vi "Bodies_GetPtJacobian.vi"(8 "error in (no error)":errorcluster, 10 "Point":T1, 11 "Bodies.lvclass":refnum<class "Bodies.lvclass">) -> (0 "error out":errorcluster, 1 "PointInGCS":dbl[](array[numeric]) format="%#.6f", 2 "Jacobian":dbl[][](array[numeric]) format="%#.6f", 3 "Bodies.lvclass 2":refnum<class "Bodies.lvclass">)   [LabVIEW 2015, in "Bodies.lvclass"]
doc: "Calculate velocity Jacobian v=[J] dq. Input the point of interest (POI) in local coordinate system. Output the Jacobian that transfers the joint speed to the POI's speed."
uses:
  Bodies.lvclass
  PointOnBody.ctl
  Bodies.lvclass/Bodies.ctl
  xyzO.ctl
  <vilib>/Analysis/NI_AALPro.lvlib
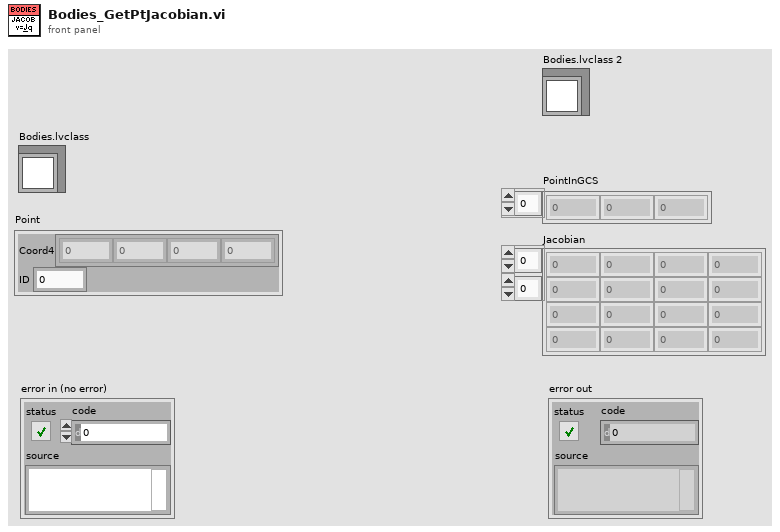
[diagram p1: front panel]
types:
  T1 = typedef "Bodies.lvclass/PointOnBody.ctl" = cluster{"Coord4":dbl[], "ID":i32}
  T2 = typedef "Bodies.lvclass/xyzO.ctl" = enum16{"X", "Y", "Z", "O"}
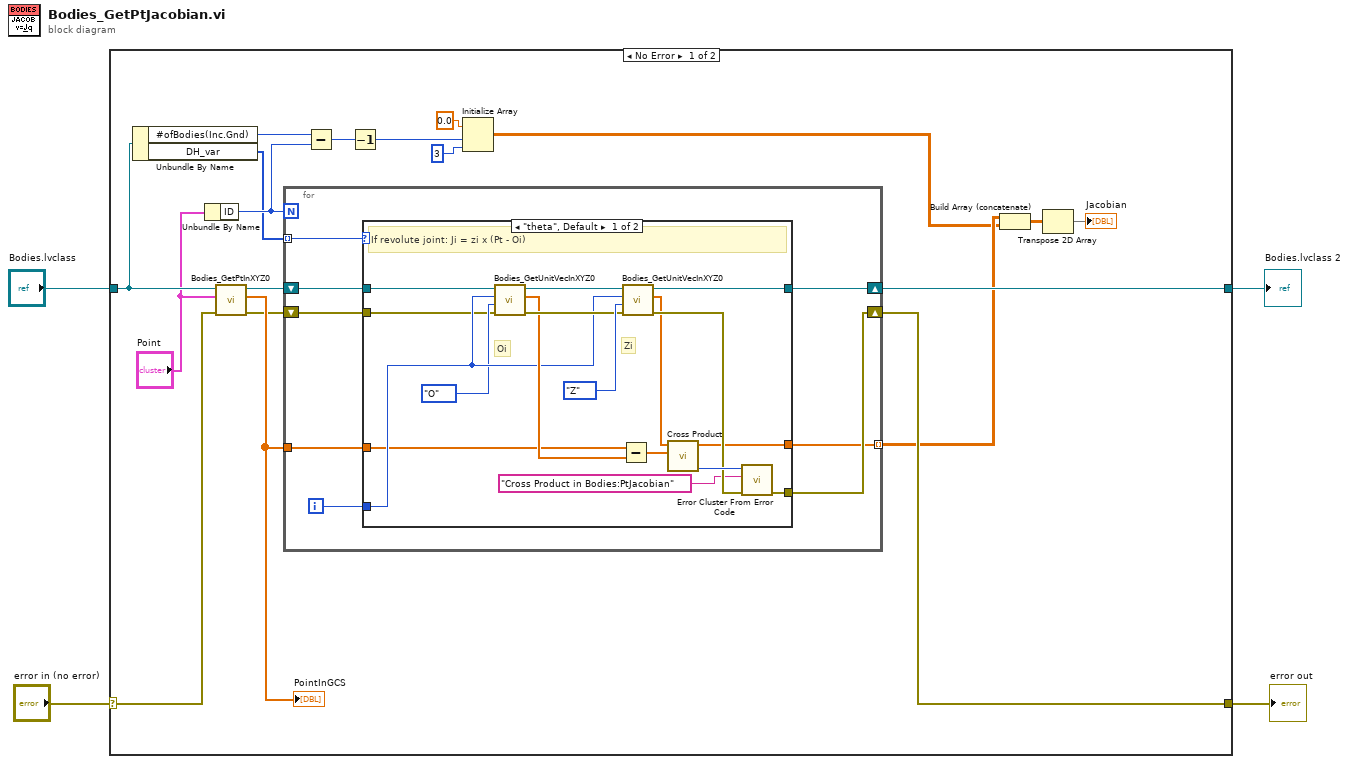
[diagram p0: block diagram]
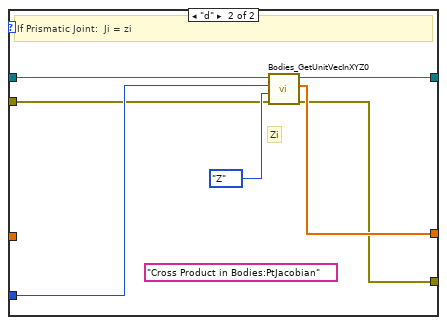
[diagram p2: hidden frame]
diagram:
  n1 = case shown="No Error" "error in (no error)" {
    selector: "error in (no error)" -> [w7 w57]
    tunnel: "Bodies.lvclass" -> [w11 w56]
    tunnel: [w23 w57] -> w3
    tunnel: [w22 w56] -> w2
    frame No Error {
      n2 = Unbundle By Name(w11) -> ("#ofBodies(Inc.Gnd)"=w21:i32, "DH_var"=w5:enum16{"theta", "d"}[])
      n3 = Unbundle By Name("Point") -> ("ID"=w20:i32)
      n4 = call "Bodies_GetPtInXYZ0.vi"("error in (no error)"=w7, "Point"="Point", "Bodies.lvclass"=w11) -> ("error out"=w6:errorcluster, "PointInGCS"=w8:dbl[], "Bodies.lvclass 2"=w10:refnum<class "Bodies.lvclass">)  [unwired: 5 in, 1 out]
      "PointInGCS" <- w8
      n5 = for {
        N: w20 -> [_]
        shift-right: [w29] -> w23
        shift-left: w6 -> [w26]
        shift-right: [w31] -> w22
        shift-left: w10 -> [w25]
        tunnel: [w28] -> w16 mode=indexing
        tunnel: w8 -> [w27]
        tunnel: w5 -> [w24] mode=indexing
        i -> [w30]
        n6 = case shown="\"theta\", Default" w24 {
          tunnel: [w48 w55] -> w31
          tunnel: w30 -> [w41 w53]
          tunnel: [w39 w49] -> w29
          tunnel: [w36 w50] -> w28
          tunnel: w27 -> [w35 _]
          tunnel: w26 -> [w34 w51]
          tunnel: w25 -> [w32 w52]
          frame "theta", Default {
            # "Oi"
            # "Zi"
            # "If revolute joint: Ji = zi x (Pt - Oi)"
            n7 = call "Bodies_GetUnitVecInXYZ0.vi"("error in (no error)"=w34, "Dir of Vector"=xyzO."O" ("Dir"), "Body ID"=w41, "Bodies.lvclass"=w32) -> ("error out"=w43:errorcluster, "UnitVec in GCS"=w42:dbl[], "Bodies.lvclass 2"=w44:refnum<class "Bodies.lvclass">)  [unwired: 5 in]
            n8 = Subtract(x=w35, y=w42) -> (x-y=w37:dbl[])
            n9 = call "Bodies_GetUnitVecInXYZ0.vi"("error in (no error)"=w43, "Dir of Vector"=xyzO."Z" ("Dir"), "Body ID"=w41, "Bodies.lvclass"=w44) -> ("error out"=w45:errorcluster, "UnitVec in GCS"=w38:dbl[], "Bodies.lvclass 2"=w48:refnum<class "Bodies.lvclass">)  [unwired: 5 in]
            n10 = call <vilib>:"Cross Product.vi"("B Vector"=w37, "A Vector"=w38) -> ("error"=w46:i32, "Cross Product"=w36:dbl[])  [unwired: 8 in]
            n11 = call <vilib>:"Error Cluster From Error Code.vi"("error in (no error)"=w45, "error message (\"\")"="Cross Product in Bodies:PtJacobian" ("error source (\" \")"), "error code (0)"=w46) -> ("error out"=w39:errorcluster)  [unwired: 6 in]
          }
          frame "d" {
            (unwired) "Cross Product in Bodies:PtJacobian" ("error source (\" \")")
            # "Zi"
            # "If Prismatic Joint:  Ji = zi"
            n12 = call "Bodies_GetUnitVecInXYZ0.vi"("error in (no error)"=w51, "Dir of Vector"=xyzO."Z" ("Dir"), "Body ID"=w53, "Bodies.lvclass"=w52) -> ("error out"=w49:errorcluster, "UnitVec in GCS"=w50:dbl[], "Bodies.lvclass 2"=w55:refnum<class "Bodies.lvclass">)  [unwired: 5 in]
          }
        }
      }
      n13 = Subtract(x=w21, y=w20) -> (x-y=w17:i32)
      n14 = Decrement(x=w17) -> (x-1=w14:i32)
      n15 = Initialize Array(0.0 ("element"), w14, 3 ("dimension size")) -> (w15:dbl[][])
      n16 = Build Array (concatenate)(w16, w15) -> (w18:dbl[][])
      n17 = Transpose 2D Array(2D array=w18) -> (transposed array=→"Jacobian":dbl[][])
    }
    frame Error {
    }
  }
  "error out" <- w3
  "Bodies.lvclass 2" <- w2
